vi "CreateResultTreeListener_WithResultTree_ReturnsNoError.vi"() -> (0 "error out":errorcluster)   [LabVIEW 2017, in "ResultTreeListener.Tests.lvlib"]
uses:
  ResultTreeListener.Tests.lvlib
  ResultTreeListener/ResultTreeListener.lvclass
  Assertion/Assertion.lvlib
  ResultTree/ResultTree.lvclass
panel:
  in  "Tree":string(tree)
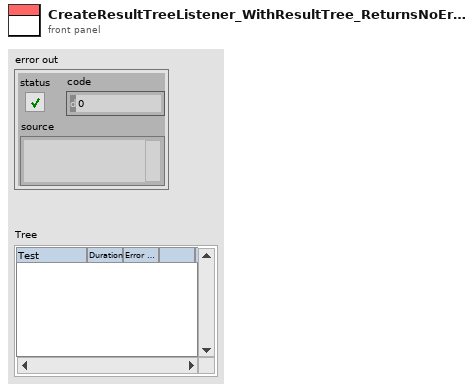
[diagram p1: front panel]
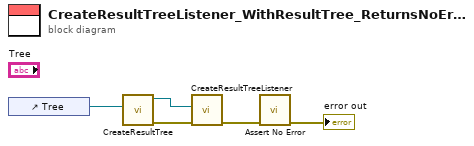
[diagram p0: block diagram]
diagram:
  n1 = control-ref of="Tree"() -> (w3:refnum<vi>)
  n2 = call "CreateResultTree.vi"("Tree Refnum"=w3) -> ("error out"=w5:errorcluster, "ResultTree out"=w4:refnum<class "ResultTree.lvclass">)  [unwired: 9 in]
  n3 = call "CreateResultTreeListener.vi"("error in (no error)"=w5, "ResultTree"=w4) -> ("error out"=w2:errorcluster)  [unwired: 8 in, 1 out]
  n4 = call "Assert No Error.vi"("error in (no error)"=w2) -> ("error out"=→"error out":errorcluster)  [unwired: 10 in]
